vi "BtnPress.vi"(0 "queue in":refnum<queue>, 2 "CtlRef":refnum<vi>, 7 "Msg":string, 11 "error in":errorcluster) -> (4 "queue out":refnum<queue>, 15 "error out":errorcluster)   [LabVIEW 2026]
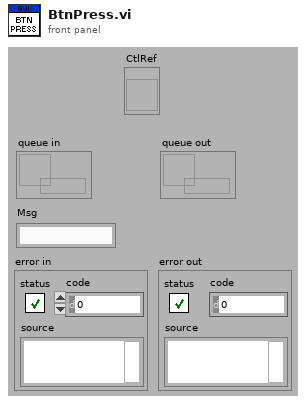
[diagram p1: front panel]
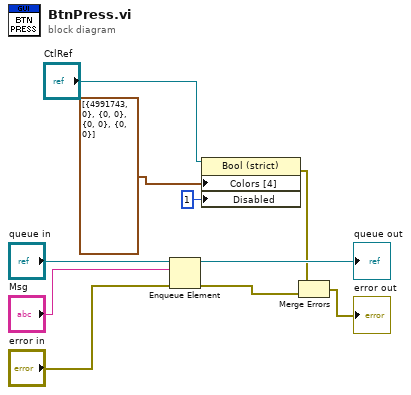
[diagram p0: block diagram]
diagram:
  n1 = Enqueue Element(queue="queue in", element="Msg", error in (no error)="error in") -> (queue out=→"queue out":refnum<queue>, error out=w3:errorcluster)  [unwired: 1 in, 1 out]
  n2 = property class="Bool (strict)"(reference="CtlRef", "Colors [4]"=cluster{u32, u32}[] [{4991743, 0}, {0, 0}, {0, 0}, {0, 0}], "Disabled"=u8 1) -> (error out=w4:errorcluster)  [unwired: 1 in, 1 out]
  n3 = Merge Errors(w4, w3) -> (→"error out":errorcluster)
